vi "getTopic.vi"(8 "error in (no error)":errorcluster, 10 "Alias":string, 11 "DICT in":refnum<class "DICT.lvclass">) -> (0 "error out":errorcluster, 1 "TopicFound":bool, 2 "Topic":string, 3 "DICT out":refnum<class "DICT.lvclass">)   [LabVIEW 2017, in "DICT.lvclass"]
uses:
  DICT.lvclass
  DICT.lvclass/DICT.ctl
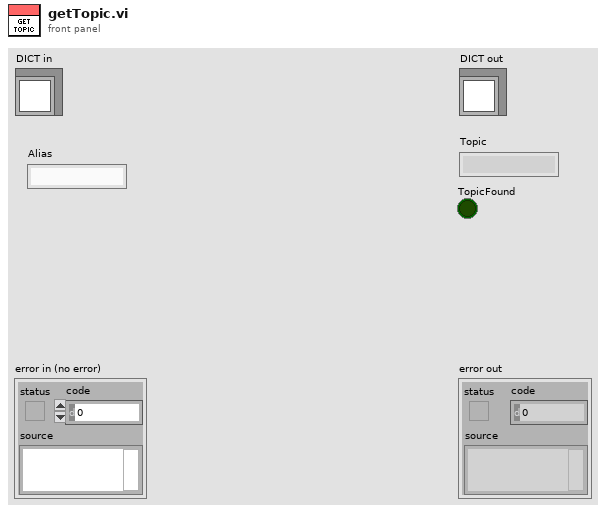
[diagram p1: front panel]
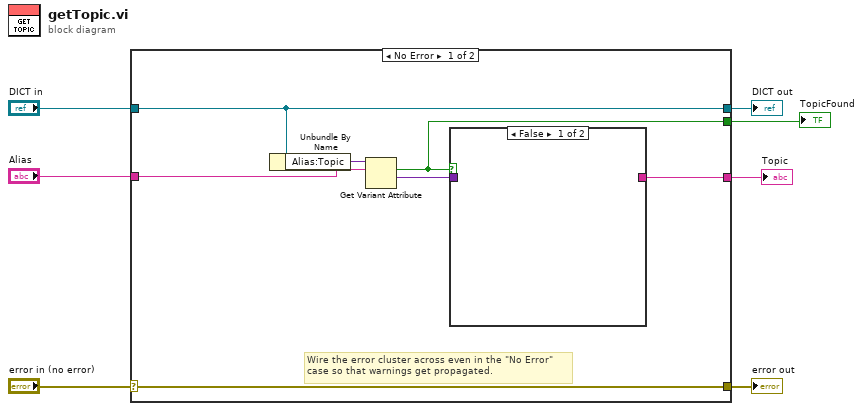
[diagram p0: block diagram]
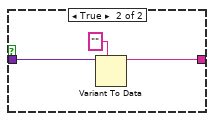
[diagram p2: hidden frame]
diagram:
  n1 = case shown="No Error" "error in (no error)" {
    selector: "error in (no error)" -> [w14 w19]
    tunnel: [w14 w19] -> w6
    tunnel: [w13 w18] -> w4
    tunnel: "DICT in" -> [w13 w18]
    tunnel: "Alias" -> [w11 _]
    tunnel: [w9 _] -> w2
    tunnel: [w8 _] -> w1
    frame No Error {
      # "Wire the error cluster across even in the \"No Error\"\ncase so that warnings get propagated."
      n2 = Unbundle By Name(w13) -> ("Alias:Topic"=w12:variant)
      n3 = Get Variant Attribute(Variant=w12, name=w11) -> (found=w8:bool, value=w10:variant)  [unwired: 2 in, 2 out]
      n4 = case shown="False" w8 {
        tunnel: w10 -> [_ w17]
        tunnel: [_ w15] -> w9
        frame False {
        }
        frame True {
          n5 = Variant To Data(type="" ("Topic"), Variant=w17) -> (data=w15:string)  [unwired: 1 in, 1 out]
        }
      }
    }
    frame Error {
    }
  }
  "error out" <- w6
  "DICT out" <- w4
  "Topic" <- w2
  "TopicFound" <- w1
